vi "Destroy.vi"(0 "Suggestion IO in":refnum<class "SuggestionIObase.lvclass">, 11 "error in (no error)":errorcluster) -> (4 "Suggestion IO out":refnum<class "SuggestionIObase.lvclass">, 15 "error out":errorcluster)   [LabVIEW 2016, in "SuggestionIObase.lvclass"]
uses:
  SuggestionIObase.lvclass
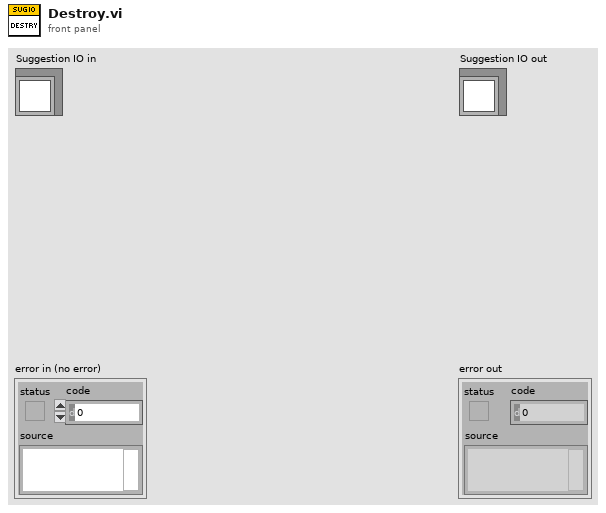
[diagram p1: front panel]
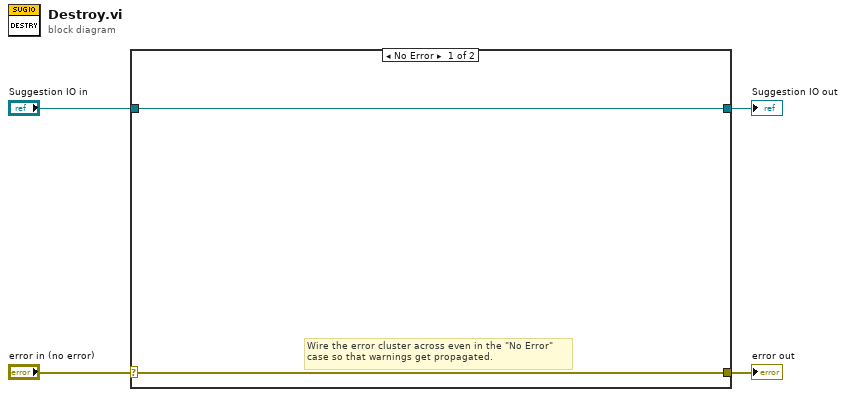
[diagram p0: block diagram]
diagram:
  n1 = case shown="No Error" "error in (no error)" {
    selector: "error in (no error)" -> [w5 w8]
    tunnel: [w5 w8] -> w3
    tunnel: [w6 w7] -> w1
    tunnel: "Suggestion IO in" -> [w6 w7]
    frame No Error {
      # "Wire the error cluster across even in the \"No Error\"\ncase so that warnings get propagated."
    }
    frame Error {
    }
  }
  "error out" <- w3
  "Suggestion IO out" <- w1
